vi "NI9215_scaler.vi"() -> ()   [LabVIEW 2019]
uses:
  <vilib>/Platform/TimedLoop/XDataNode/timing_clust.ctl
  <vilib>/Platform/TimedLoop/XDataNode/nitl_modes.ctl
  <vilib>/Platform/TimedLoop/XDataNode/wakeup.ctl
  <vilib>/rvi/Emulation/niFpgaGetClockAttributes.vi
  <vilib>/rvi/Emulation/niFpgaSctlEmulationGetInTimedLoop.vi
  <vilib>/rvi/Emulation/niFpgaEmulationReportErrorSimple.vi
  <vilib>/rvi/Emulation/niFpgaCriticalErrorInLSC.vi
  <vilib>/rvi/Emulation/niFpgaProcessEmulError.vi
  <vilib>/rvi/eio/common/nirviEmuTemplateMethod_errors.vi
  <vilib>/platform/TimedLoop/XDataNode/XDataNode.xnode
  <vilib>/eio/EIONode/EIONode.xnode
  <vilib>/Platform/TimedLoop/XDataNode/XDNodeRunTimeDep.lvlib
  lib/Scaler-EPICS/scaler.lvlib
panel:
  in  "Enable_SCALER 2":bool
  in  "OneShot_SCALER 2":bool
  in  "SampleAnalog_SCALER 2":bool
  in  "Gate_SCALER 2":bool[](array[boolean])=[FALSE, FALSE, FALSE, FALSE, FALSE]
  in  "PresetValues_SCALER 2":u32[](array[numeric])=[0, 0, 0, 0, 0]
  in  "fxp_ShiftLeft_SCALER 2":u64
  out "Done_SCALER 2":bool
  out "fxp_AnalogOutput0_SCALER 2":u64
  out "fxp_AnalogOutput1_SCALER 2":u64
  out "fxp_AnalogOutput2_SCALER 2":u64
  out "fxp_AnalogOutput3_SCALER 2":u64
  out "Counter_SCALER 2":u32[](array[numeric])
  out "AnalogInputs_Scaler 2":fxp<+/-,20,5>[](array[numeric]) format="%.17g"
  out "Looptime 2":u32
  out "Counter_SCALER":u32[](array[numeric])
  out "fxp_AnalogOutput3_SCALER":u64
  out "fxp_AnalogOutput2_SCALER":u64
  out "fxp_AnalogOutput1_SCALER":u64
  out "fxp_AnalogOutput0_SCALER":u64
  out "Done_SCALER":bool
  in  "fxp_ShiftLeft_SCALER":u64
  in  "PresetValues_SCALER":u32[](array[numeric])=[0, 0, 0, 0, 0]
  in  "Gate_SCALER":bool[](array[boolean])=[FALSE, FALSE, FALSE, FALSE, FALSE]
  in  "SampleAnalog_SCALER":bool
  in  "OneShot_SCALER":bool
  in  "Enable_SCALER":bool
  out "Looptime":u32
  out "AnalogInputs_Scaler":fxp<+/-,20,5>[](array[numeric]) format="%.17g"
  # "Optimization tip:\nMake all the arrays the same size as the number\nof channels you need implemented. Setting\nthe number of channels uses up to 60% of the \nresources. Setting to 2 uses only 27%."
  # "This is a 2 channel analog scaler. It follows to the word the definition of the scaler in the anl website\nhttps://epics.anl.gov/bcda/synApps/std/scalerRecord.html"
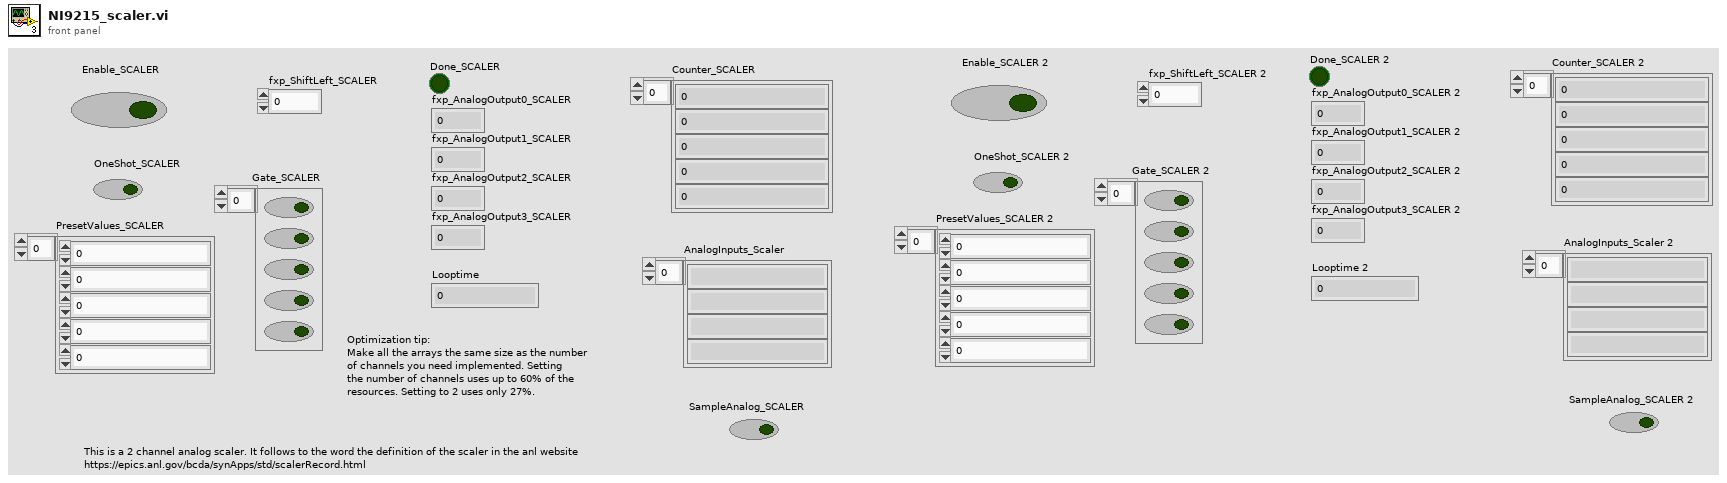
[diagram p1: front panel]
types:
  T1 = typedef "XDNodeRunTimeDep.lvlib/timing_clust.ctl" = cluster{"Expected End [f-1]":u64, "Actual End [f-1]":u64, "Finished Late? [f-1]":bool, "Expected End [i-1]":u64, "Actual End [i-1]":u64, "Finished Late? [i-1]":bool, "Expected Start [i]":u64, "Actual Start [i]":u64, "Expected Start [f]":u64, "Actual Start [f]":u64, "Source Name":string, "Structure Name":string, "Period":i64, "Deadline":i64, "Offset":i64, "Start":i64, "Priority":i32, "Timeout":i32, "Mode":T2, "Wakeup Reason":T3, "Error":errorcluster, "Source Type":string, "Secondary Source Type":string, "Global End Time":u64, "Global Start Time":u64, "Frame Duration":u64, "Iteration Duration":u64, "Assigned CPU":i32, "I/O Scan Engine Mode":u32}
  T2 = typedef "XDNodeRunTimeDep.lvlib/nitl_modes.ctl" = enum32{"No Change", "Process missed periods, maintain original phase", "Discard missed periods, maintain original phase", "Process missed periods, ignore original phase", "Discard missed periods, ignore original phase"}
  T3 = typedef "XDNodeRunTimeDep.lvlib/wakeup.ctl" = enum32{"Normal", "Aborted", "Asynchronous wakeup", "Timing source error", "Timed loop error", "Timeout"}
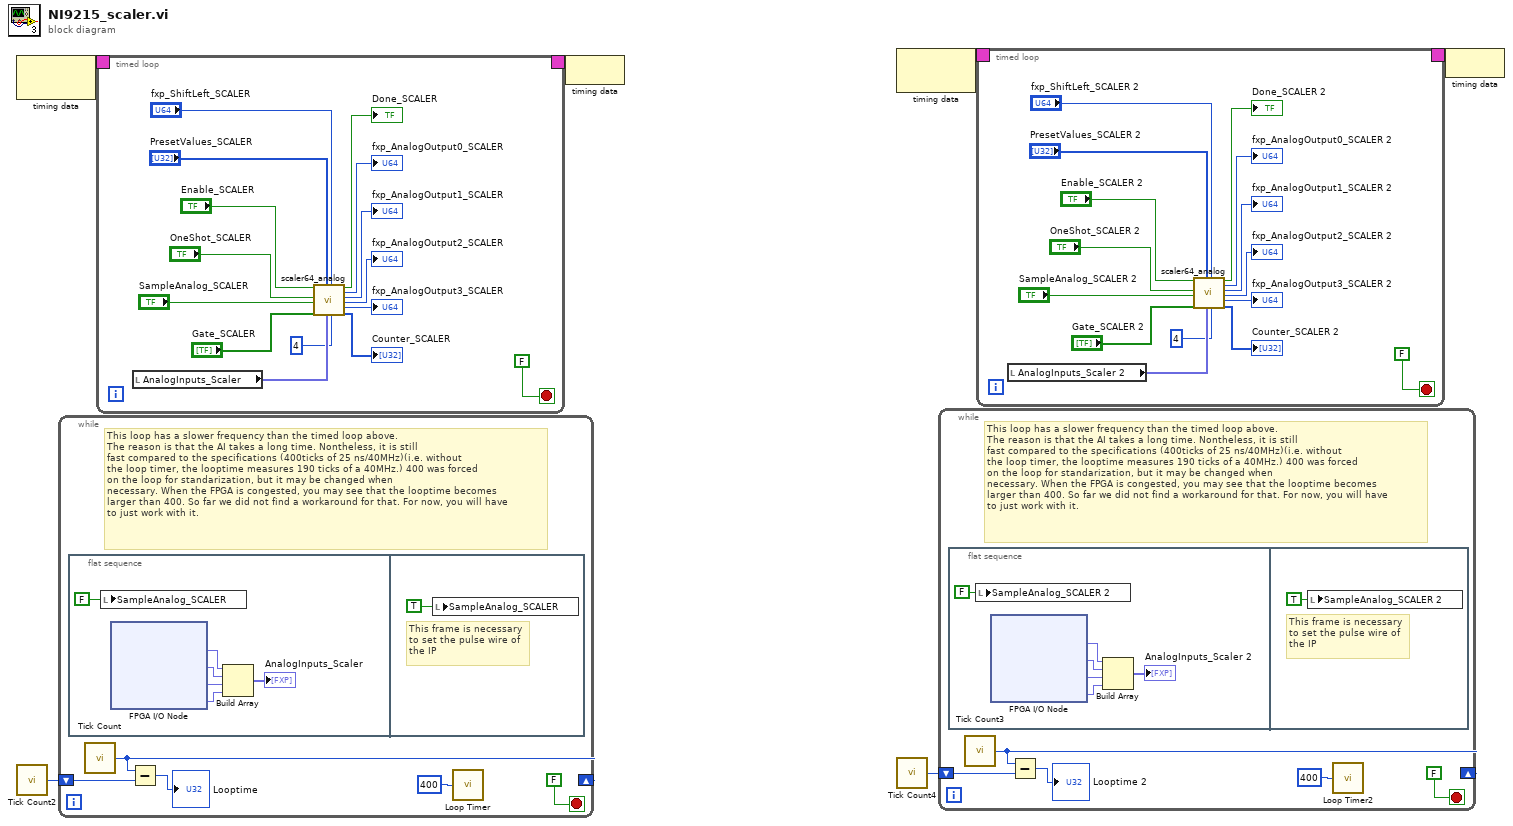
[diagram p0: block diagram]
diagram:
  n1 = node-c288() -> (w6:T1)  [unwired: 1 in]
  n2 = call "Tick Count2"() -> ("Tick Count(Ticks)"=w4:u32)
  n3 = while {
    shift-right: [w8] -> _
    shift-left: w4 -> [w9]
    stop <- FALSE stop-if-true
    # "This loop has a slower frequency than the timed loop above.\nThe reason is that the AI takes a long time. Nontheless, it is still\nfast compared to the specifications (400ticks of 25 ns/40MHz)(i.e. without \nthe loop timer, the looptime measures 190 ticks of a 40MHz.) 400 was forced \non the loop for standarization, but it may be changed when \nnecessary. When the FPGA is congested, you may see that the looptime becomes \nlarger than 400. So far we did not find a workaround for that. For now, you will have\nto just work with it."
    n4 = flat-sequence {
      frame #0 {
        n5 = local write "SampleAnalog_SCALER"(FALSE) -> ()
        n6 = xnode "FPGA I/O Node"() -> ("Mod4/AI0"=w17:fxp<+/-,20,5>, "Mod4/AI1"=w15:fxp<+/-,20,5>, "Mod4/AI2"=w14:fxp<+/-,20,5>, "Mod4/AI3"=w13:fxp<+/-,20,5>)  [unwired: 4 in, 4 out]
        n7 = Build Array(w17, w15, w14, w13) -> (→"AnalogInputs_Scaler":fxp<+/-,20,5>[])
      }
      frame #1 {
        # "This frame is necessary to set the pulse wire of the IP"
        n8 = local write "SampleAnalog_SCALER"(TRUE ("sample")) -> ()
      }
    }
    n9 = call "Tick Count"() -> ("Tick Count(Ticks)"=w8:u32)
    n10 = Subtract(x=w8, y=w9) -> (x-y=→"Looptime":u32)
    n11 = call "Loop Timer"("Count(Ticks)"=i16 400) -> ()  [unwired: 1 out]
  }
  n12 = timed-loop {
    timing: w6 -> [_]
    timing-out: [_] -> w5
    stop <- FALSE stop-if-true
    n13 = local read "AnalogInputs_Scaler"() -> (w32:fxp<+/-,20,5>[])
    n14 = call "scaler64_analog.vi"("Enable_SCALER"="Enable_SCALER", "OneShot_SCALER"="OneShot_SCALER", "SampleAnalog_SCALER"="SampleAnalog_SCALER", "Gate_SCALER"="Gate_SCALER", "PresetValues_SCALER"="PresetValues_SCALER", "AnalogInputs_SCALER"=w32, "fxp_ShiftLeft_SCALER"="fxp_ShiftLeft_SCALER", "divisor_SCALER"=i16 4) -> ("Done_SCALER"=→"Done_SCALER":bool, "fxp_RawAI0_SCALER"=→"fxp_AnalogOutput0_SCALER":u64, "fxp_RawAI1_SCALER"=→"fxp_AnalogOutput1_SCALER":u64, "fxp_RawAI2_SCALER"=→"fxp_AnalogOutput2_SCALER":u64, "fxp_RawAI3_SCALER"=→"fxp_AnalogOutput3_SCALER":u64, "Counter_SCALER"=→"Counter_SCALER":u32[])  [unwired: 5 in, 1 out]
  }
  n15 = node-c288(w5) -> ()
  n16 = node-c288() -> (w3:T1)  [unwired: 1 in]
  n17 = call "Tick Count4"() -> ("Tick Count(Ticks)"=w1:u32)
  n18 = while {
    shift-right: [w37] -> _
    shift-left: w1 -> [w38]
    stop <- FALSE stop-if-true
    # "This loop has a slower frequency than the timed loop above.\nThe reason is that the AI takes a long time. Nontheless, it is still\nfast compared to the specifications (400ticks of 25 ns/40MHz)(i.e. without \nthe loop timer, the looptime measures 190 ticks of a 40MHz.) 400 was forced \non the loop for standarization, but it may be changed when \nnecessary. When the FPGA is congested, you may see that the looptime becomes \nlarger than 400. So far we did not find a workaround for that. For now, you will have\nto just work with it."
    n19 = flat-sequence {
      frame #0 {
        n20 = local write "SampleAnalog_SCALER 2"(FALSE) -> ()
        n21 = xnode "FPGA I/O Node"() -> ("Mod7/AI0"=w46:fxp<+/-,20,5>, "Mod7/AI1"=w44:fxp<+/-,20,5>, "Mod7/AI2"=w43:fxp<+/-,20,5>, "Mod7/AI3"=w42:fxp<+/-,20,5>)  [unwired: 4 in, 4 out]
        n22 = Build Array(w46, w44, w43, w42) -> (→"AnalogInputs_Scaler 2":fxp<+/-,20,5>[])
      }
      frame #1 {
        # "This frame is necessary to set the pulse wire of the IP"
        n23 = local write "SampleAnalog_SCALER 2"(TRUE ("sample")) -> ()
      }
    }
    n24 = call "Tick Count3"() -> ("Tick Count(Ticks)"=w37:u32)
    n25 = Subtract(x=w37, y=w38) -> (x-y=→"Looptime 2":u32)
    n26 = call "Loop Timer2"("Count(Ticks)"=i16 400) -> ()  [unwired: 1 out]
  }
  n27 = timed-loop {
    timing: w3 -> [_]
    timing-out: [_] -> w2
    stop <- FALSE stop-if-true
    n28 = local read "AnalogInputs_Scaler 2"() -> (w61:fxp<+/-,20,5>[])
    n29 = call "scaler64_analog.vi"("Enable_SCALER"="Enable_SCALER 2", "OneShot_SCALER"="OneShot_SCALER 2", "SampleAnalog_SCALER"="SampleAnalog_SCALER 2", "Gate_SCALER"="Gate_SCALER 2", "PresetValues_SCALER"="PresetValues_SCALER 2", "AnalogInputs_SCALER"=w61, "fxp_ShiftLeft_SCALER"="fxp_ShiftLeft_SCALER 2", "divisor_SCALER"=i16 4) -> ("Done_SCALER"=→"Done_SCALER 2":bool, "fxp_RawAI0_SCALER"=→"fxp_AnalogOutput0_SCALER 2":u64, "fxp_RawAI1_SCALER"=→"fxp_AnalogOutput1_SCALER 2":u64, "fxp_RawAI2_SCALER"=→"fxp_AnalogOutput2_SCALER 2":u64, "fxp_RawAI3_SCALER"=→"fxp_AnalogOutput3_SCALER 2":u64, "Counter_SCALER"=→"Counter_SCALER 2":u32[])  [unwired: 5 in, 1 out]
  }
  n30 = node-c288(w2) -> ()
